vi "GetCurrentPosition.vi"(8 "error in (no error)":errorcluster, 11 "Serial Controller in":refnum<class "Serial Controller.lvclass">) -> (0 "error out":errorcluster, 2 "Position":dbl[](array[numeric]), 3 "Serial Controller out":refnum<class "Serial Controller.lvclass">)   [LabVIEW 2010, in "Serial Controller.lvclass"]
uses:
  Serial Controller.lvclass
  Serial Controller.lvclass/Serial Controller.ctl
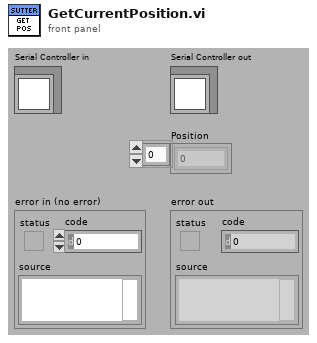
[diagram p1: front panel]
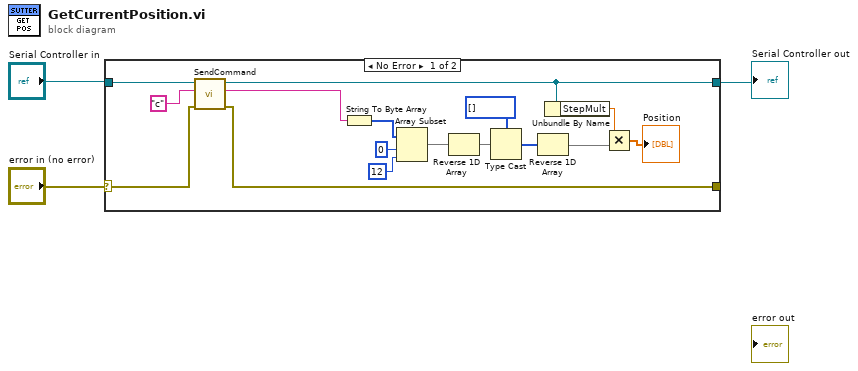
[diagram p0: block diagram]
diagram:
  n1 = case shown="No Error" "error in (no error)" {
    selector: "error in (no error)" -> [w10 w21]
    tunnel: [w9 w21] -> _
    tunnel: [w7 w20] -> w2
    tunnel: "Serial Controller in" -> [w12 w20]
    frame No Error {
      n2 = call-dynamic "SendCommand.vi"("error in (no error)"=w10, "command"="c", "Serial Controller in"=w12) -> ("error out"=w9:errorcluster, "Returned"=w8:string, "Serial Controller out"=w7:refnum<class "Serial Controller.lvclass">)  [unwired: 6 in]
      n3 = String To Byte Array(string=w8) -> (unsigned byte array=w19:u8[])
      n4 = Array Subset(array=w19, index=0, length=12) -> (w15:u8[])
      n5 = Reverse 1D Array(array=w15) -> (reversed array=w14:u8[])
      n6 = Type Cast(type=i32[] [], x=w14) -> (*(type *) &x=w13:i32[])
      n7 = Reverse 1D Array(array=w13) -> (reversed array=w6:i32[])
      n8 = Unbundle By Name(w7) -> ("StepMult"=w5:dbl)
      n9 = Multiply(x=w5, y=w6) -> (x*y=→"Position":dbl[])
    }
    frame Error {
    }
  }
  "Serial Controller out" <- w2
